vi "Period Curve from Matrix Signals.vi"(5 "S-G Polynomial Order":i32=3, 6 "Interpolation Method":i32(ring)=2 items=["nearest", "linear", "spline", "cubic Hermite", "Lagrange"], 7 "S-G Side Points":i32=15, 9 "first_discard_bins":dbl=100.0, 11 "Signals Matrix":T1) -> (0 "Not-Extended Period Length Curve":cluster{"yi":dbl[], "yi":dbl[]}(graph), 2 "Period Length Curve by  Fitting":dbl[](graph), 3 "Period Length Curve by Interpolation":dbl[](graph))   [LabVIEW 2014]
uses:
  <vilib>/Analysis/Matrix/Datatypes/RealMatrix.ctl
  <vilib>/Analysis/3filter.llb/Savitzky-Golay Filter (DBL).vi
  <vilib>/imath/engines/lvmath2/RunTimeEngine/RangeToken/NIMS_Range.vi
  <instcachedir>/0/NIMS_Range_9BCE657718DF4976A877346C61F22738.lvgen/NIMS_Range_9BCE657718DF4976A877346C61F22738_001.vi
  <vilib>/imathl/engines/lvmath/Functions/Error Handling/Create Error.vi
  <vilib>/imath/engines/lvmath2/RunTimeEngine/BuiltInFunctions/polyfit/NIMS_[2o]_polyfit.vi
  <vilib>/imath/engines/lvmath2/RunTimeEngine/ErrorHandling/NIMS_Error From Error Code.vi
  <vilib>/imath/engines/lvmath2/RunTimeEngine/BuiltInFunctions/polyval/NIMS_polyval(GV,GM).vi
  <instcachedir>/0/NIMS_polyval(GV,GM)_E12556DC54744E0C81968744501C4F35.lvgen/NIMS_polyval(GV,GM)_E12556DC54744E0C81968744501C4F35_002.vi
  <vilib>/imath/engines/lvmath2/RunTimeEngine/ArithmeticOperatorToken/NIMS_ArithmeticOperator_minus.vi
  <instcachedir>/0/NIMS_ArithmeticOperator_minus_39C0593E74DA4138ACA2AB742906488D.lvgen/NIMS_ArithmeticOperator_minus_39C0593E74DA4138ACA2AB742906488D_003.vi
  <vilib>/imath/engines/lvmath2/RunTimeEngine/NodeEndStatement/NIMS_NodeEndStatement_Output.vi
  <instcachedir>/0/NIMS_NodeEndStatement_Output_53EC0D466D134D7ABD903AC30B43404B.lvgen/NIMS_NodeEndStatement_Output_53EC0D466D134D7ABD903AC30B43404B_005.vi
  <vilib>/imath/engines/lvmath2/RunTimeEngine/ErrorHandling/NIMS_Finalize Error.vi
  <vilib>/imath/engines/lvmath2/RunTimeEngine/BuiltInFunctions/round/NIMS_round(DBL-V).vi
  <vilib>/imath/engines/lvmath2/RunTimeEngine/BuiltInFunctions/difference/NIMS_difference(GV,I32).vi
  <instcachedir>/0/NIMS_difference(GV,I32)_DC7351DCBCF840A8AE147F50EC2CE86E.lvgen/NIMS_difference(GV,I32)_DC7351DCBCF840A8AE147F50EC2CE86E_000.vi
  <vilib>/imath/engines/lvmath2/RunTimeEngine/BuiltInFunctions/size/NIMS_I32=size(GCol,I32).vi
  <instcachedir>/0/NIMS_I32=size(GCol,I32)_E76181316ED84D3E8F11BE44C7815EB0.lvgen/NIMS_I32=size(GCol,I32)_E76181316ED84D3E8F11BE44C7815EB0_000.vi
  <vilib>/imath/engines/lvmath2/RunTimeEngine/IndexRead/NIMS V(R2).vi
  <instcachedir>/0/NIMS V(R2)_C76619605A0E4E9F8B2FA9389712AC47.lvgen/NIMS V(R2)_C76619605A0E4E9F8B2FA9389712AC47_000.vi
  <vilib>/imath/engines/lvmath2/RunTimeEngine/ErrorHandling/NIMS_Create Error From Enums.vi
  <vilib>/imath/engines/lvmath2/RunTimeEngine/BuiltInFunctions/zeros/NIMS_M=zeros(I32).vi
  <vilib>/imath/engines/lvmath2/RunTimeEngine/RangeToken/NIMS_Range_R2 - Integer.vi
  <instcachedir>/0/NIMS_Range_R2 - Integer_2D1304BAF97744E0A293025746CBADFC.lvgen/NIMS_Range_R2 - Integer_2D1304BAF97744E0A293025746CBADFC_000.vi
  <vilib>/imath/engines/lvmath2/RunTimeEngine/CommandStatement/MC_CommandStatement_break.vi
  <vilib>/imath/engines/lvmath2/RunTimeEngine/IndexRead/NIMS V(S).vi
  <instcachedir>/0/NIMS V(S)_0488751826AF41519A22953C041130DC.lvgen/NIMS V(S)_0488751826AF41519A22953C041130DC_000.vi
  <vilib>/imath/engines/lvmath2/RunTimeEngine/IndexReplace/NIMS M(S)=S.vi
  <instcachedir>/0/NIMS M(S)=S_D871EE7B27E5455586ED06C330670F09.lvgen/NIMS M(S)=S_D871EE7B27E5455586ED06C330670F09_001.vi
  <vilib>/imath/engines/lvmath2/RunTimeEngine/IndexRead/NIMS M($,S).vi
  <instcachedir>/0/NIMS M($,S)_3E5749BBB62E49528D4765A77F1F6D98.lvgen/NIMS M($,S)_3E5749BBB62E49528D4765A77F1F6D98_000.vi
  <vilib>/imath/engines/lvmath2/RunTimeEngine/BuiltInFunctions/zeros/NIMS_M=zeros(I32,I32).vi
  <vilib>/imath/engines/lvmath2/RunTimeEngine/IndexRead/NIMS M(S,$).vi
  <instcachedir>/0/NIMS M(S,$)_F24F360562DE41D8BE234322A2E15C65.lvgen/NIMS M(S,$)_F24F360562DE41D8BE234322A2E15C65_000.vi
  <vilib>/imath/engines/lvmath2/RunTimeEngine/BuiltInFunctions/size/NIMS_I32=size(GRow,I32).vi
  <instcachedir>/0/NIMS_I32=size(GRow,I32)_4662369BBD5B4B51BF0F6B31B2927178.lvgen/NIMS_I32=size(GRow,I32)_4662369BBD5B4B51BF0F6B31B2927178_000.vi
  <vilib>/imath/engines/lvmath2/RunTimeEngine/BuiltInFunctions/size/NIMS_I32Row=size(GCol).vi
  <instcachedir>/0/NIMS_I32Row=size(GCol)_6F63159FA7824881BFA06400543D6D03.lvgen/NIMS_I32Row=size(GCol)_6F63159FA7824881BFA06400543D6D03_000.vi
  <vilib>/imath/engines/lvmath2/RunTimeEngine/IndexRead/NIMS M($,R2).vi
  <instcachedir>/0/NIMS M($,R2)_D9380E19261A4ADFB2D364AF6959C6EF.lvgen/NIMS M($,R2)_D9380E19261A4ADFB2D364AF6959C6EF_001.vi
  <vilib>/imath/engines/lvmath2/RunTimeEngine/ArithmeticOperatorToken/NIMS_ArithmeticOperator_plus.vi
  <instcachedir>/0/NIMS_ArithmeticOperator_plus_48D6EAACA5D645B09F7EC9C016C2DEA8.lvgen/NIMS_ArithmeticOperator_plus_48D6EAACA5D645B09F7EC9C016C2DEA8_004.vi
  <vilib>/imath/engines/lvmath2/RunTimeEngine/IndexReplace/NIMS M(S,$)=V.vi
  <instcachedir>/0/NIMS M(S,$)=V_8321FD9A786642FB877A2933E8B48D2A.lvgen/NIMS M(S,$)=V_8321FD9A786642FB877A2933E8B48D2A_000.vi
  <instcachedir>/0/NIMS_NodeEndStatement_Output_53EC0D466D134D7ABD903AC30B43404B.lvgen/NIMS_NodeEndStatement_Output_53EC0D466D134D7ABD903AC30B43404B_002.vi
  <instcachedir>/0/NIMS_Range_9BCE657718DF4976A877346C61F22738.lvgen/NIMS_Range_9BCE657718DF4976A877346C61F22738_000.vi
  <instcachedir>/0/NIMS_NodeEndStatement_Output_53EC0D466D134D7ABD903AC30B43404B.lvgen/NIMS_NodeEndStatement_Output_53EC0D466D134D7ABD903AC30B43404B_001.vi
  <vilib>/imath/engines/lvmath2/RunTimeEngine/BuiltInFunctions/vconcatmx/NIMS_vconcatmx.vi
  <instcachedir>/0/NIMS_vconcatmx_3F7EE7E265C34A1F815AF13176DC5310.lvgen/NIMS_vconcatmx_3F7EE7E265C34A1F815AF13176DC5310_000.vi
  <vilib>/Analysis/NI_AALBase.lvlib
  <vilib>/Analysis/NI_AAL_SigProc.lvlib
  <vilib>/gmath/NI_Gmath.lvlib
  <vilib>/Analysis/Matrix/NI_Matrix.lvlib
panel:
  # "Smoothing: Savitzky-Golay Parameters"
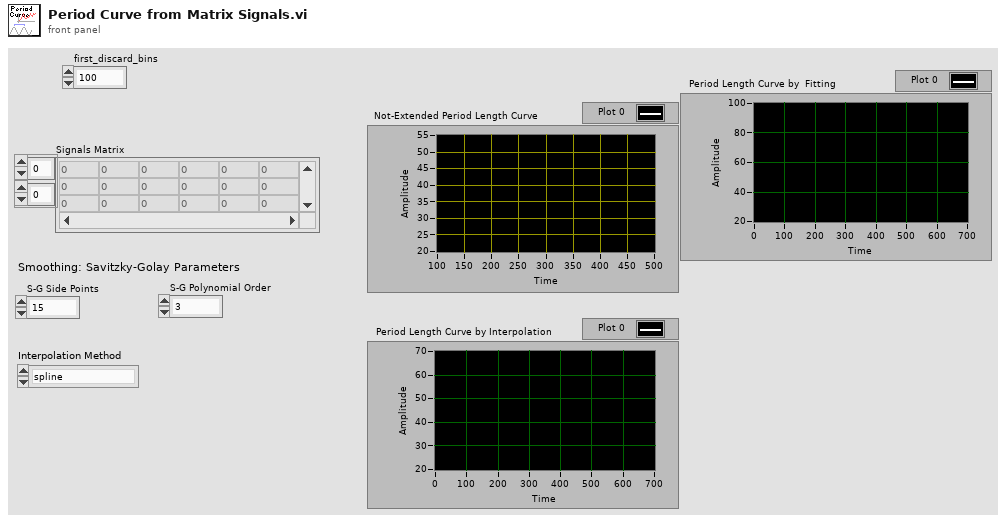
[diagram p1: front panel]
types:
  T1 = typedef "NI_Matrix.lvlib/RealMatrix.ctl" = dbl[][]
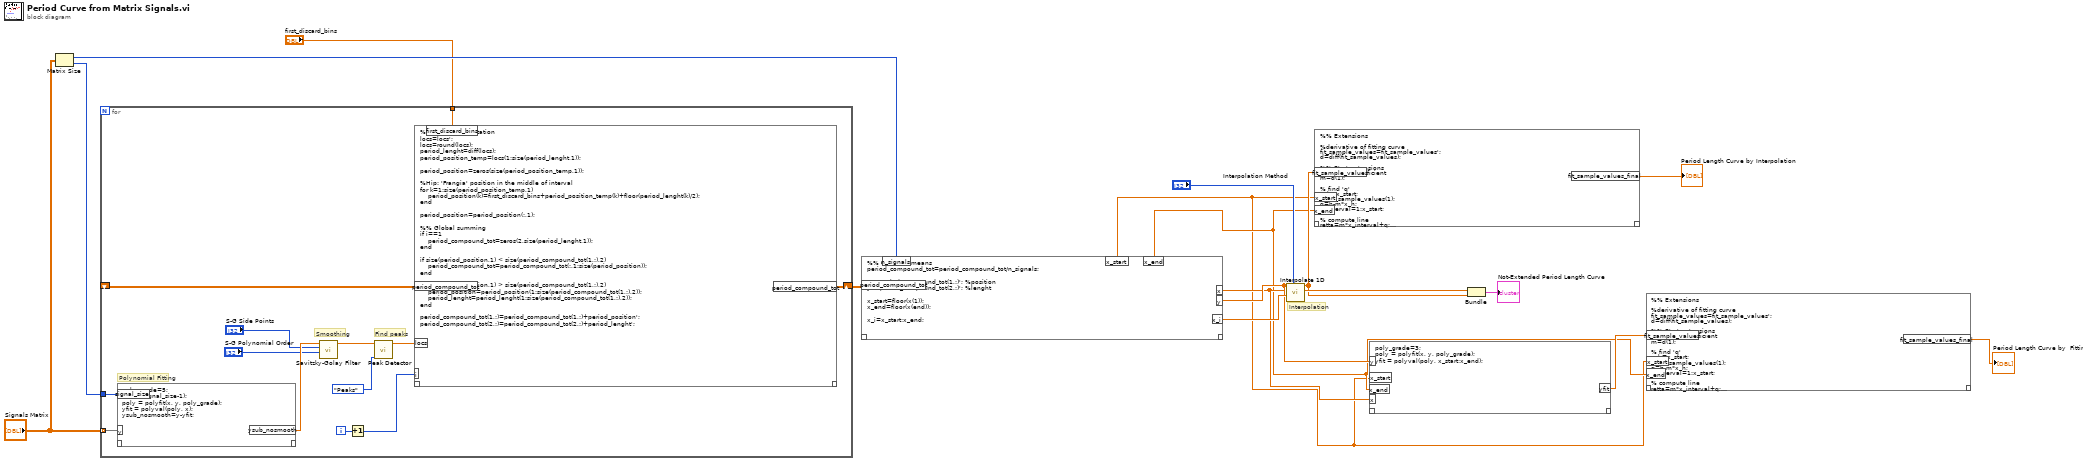
[diagram p0: block diagram]
diagram:
  # "Interpolation"
  n1 = Matrix Size(0:"Signals Matrix") -> (1:w13:i32, 2:w12:i32)
  n2 = for {
    tunnel: "Signals Matrix" -> [w26] mode=indexing
    shift-right: [w23] -> w17
    shift-left: _ -> [w22]
    tunnel: w12 -> [w21]
    tunnel: "first_discard_bins" -> [w18]
    i -> [w24]
    # "Find peaks"
    # "Smoothing"
    # "Polynomial Fitting"
    n3 = mathscript code="poly_grade=5;\nx = 0:(signal_size-1);\npoly = polyfit(x, y, poly_grade); \nyfit = polyval(poly, x); \nysub_nosmooth=y-yfit;"("signal_size"=w21, "y"=w26) -> ("ysub_nosmooth"=w30:dbl[])  [unwired: 1 in, 1 out]
    n4 = call-poly <vilib>:"Savitzky-Golay Filter.vi"("polynomial order"="S-G Polynomial Order", "side points"="S-G Side Points", "X"=w30) -> ("Filtered X"=w28:dbl[])  [unwired: 7 in, 1 out]
    n5 = Increment(x=w24) -> (x+1=w25:i32)
    n6 = call <vilib>:"Peak Detector.vi"("peaks/valleys"=enum32{"Peaks", "Valleys"}."Peaks", "X"=w28) -> ("Locations"=w27:dbl[])  [unwired: 5 in, 4 out]
    n7 = mathscript code="%% Period computation\nlocs=locs';\nlocs=round(locs);\nperiod_lenght=diff(locs);\nperiod_position_temp=locs(1:size(period_lenght,1)); \n\nperiod_position=zeros(size(period_position_temp,1));\n\n%Hip: 'Frangia' position in the middle of interval\nfor k=1:size(period_position_temp,1)\n    period_position(k)=first_discard_bins+period_position_temp(k)+floor(period_lenght(k)/2);\nend\n\nperiod_position=period_position(:,1);\n\n%% Global summing\nif i==1\n    period_compound_tot=zeros(2,size(period_lenght,1));\nend\n\nif size(period_position,1) < size(period_compound_tot(1,:),2)\n    period_compound_tot=period_compound_tot(:,1:size(period_position));\nend\n\nif size(period_position,1) > size(period_compound_tot(1,:),2)\n    period_position=period_position(1:size(period_compound_tot(1,:),2));\n    period_lenght=period_lenght(1:size(period_compound_tot(1,:),2));\nend\n\nperiod_compound_tot(1,:)=period_compound_tot(1,:)+period_position';\nperiod_compound_tot(2,:)=period_compound_tot(2,:)+period_lenght';"("locs"=w27, "first_discard_bins"=w18, "i"=w25, "period_compound_tot"=w22) -> ("period_compound_tot"=w23:dbl[][])  [unwired: 1 in, 1 out]
  }
  n8 = mathscript code="%% Compute means\nperiod_compound_tot=period_compound_tot/n_signals;\n\nx = period_compound_tot(1,:)'; %position\ny = period_compound_tot(2,:)'; %lenght\n\nx_start=floor(x(1));\nx_end=floor(x(end));\n\nx_i=x_start:x_end;"("period_compound_tot"=w17, "n_signals"=w13) -> ("x"=w5:dbl[], "y"=w6:dbl[], "x_start"=w1:dbl, "x_end"=w2:dbl, "x_i"=w7:dbl[])  [unwired: 1 in, 1 out]
  n9 = call <vilib>:"Interpolate 1D.vi"("method"="Interpolation Method", "xi"=w7, "X"=w5, "Y"=w6) -> ("xi used"=w15:dbl[], "yi"=w14:dbl[])  [unwired: 5 in, 1 out]
  n10 = mathscript code="%% Extensions\n\n%derivative of fitting curve\nfit_sample_values=fit_sample_values';\nd=diff(fit_sample_values);\n\n%% Start extensions\n% angular coefficient\nm=d(1);\n\n% find 'q'\nx_h=x_start;\nh=fit_sample_values(1);\nq=h-m*x_h;\nx_interval=1:x_start;\n\n% compute line\nretta=m*x_interval+q;\nretta=retta-(retta(end)-fit_sample_values(1));\nfit_sample_values_final=vertcat(retta(1:(end-1))',fit_sample_values);\n\n%% End extension\n% angular coefficient\nm=d(end);\n\n% find 'q'\nx_h=x_end;\nh=fit_sample_values(end);\nq=h-m*x_h;\nx_interval=x_end:625;\n\n% compute line\nretta_2=m*x_interval+q;\nretta_2=retta_2+(fit_sample_values(end)-retta_2(1));\nfit_sample_values_final=vertcat(fit_sample_values_final,retta_2(2:end)');\n\nfit_sample_values_final=fit_sample_values_final(:,1);"("fit_sample_values"=w14, "x_start"=w1, "x_end"=w2) -> ("fit_sample_values_final"=→"Period Length Curve by Interpolation":dbl[])  [unwired: 1 in, 1 out]
  n11 = mathscript code="poly_grade=3;\npoly = polyfit(x, y, poly_grade); \nyfit = polyval(poly, x_start:x_end);"("y"=w6, "x"=w5, "x_start"=w1, "x_end"=w2) -> ("yfit"=w4:dbl[])  [unwired: 1 in, 1 out]
  n12 = Bundle("xi used"=w15, "yi"=w14) -> (→"Not-Extended Period Length Curve":cluster{"xi used":dbl[], "yi":dbl[]})  [unwired: 1 in]
  n13 = mathscript code="%% Extensions\n\n%derivative of fitting curve\nfit_sample_values=fit_sample_values';\nd=diff(fit_sample_values);\n\n%% Start extensions\n% angular coefficient\nm=d(1);\n\n% find 'q'\nx_h=x_start;\nh=fit_sample_values(1);\nq=h-m*x_h;\nx_interval=1:x_start;\n\n% compute line\nretta=m*x_interval+q;\nretta=retta-(retta(end)-fit_sample_values(1));\nfit_sample_values_final=vertcat(retta(1:(end-1))',fit_sample_values);\n\n%% End extension\n% angular coefficient\nm=d(end);\n\n% find 'q'\nx_h=x_end;\nh=fit_sample_values(end);\nq=h-m*x_h;\nx_interval=x_end:625;\n\n% compute line\nretta_2=m*x_interval+q;\nretta_2=retta_2+(fit_sample_values(end)-retta_2(1));\nfit_sample_values_final=vertcat(fit_sample_values_final,retta_2(2:end)');\n\nfit_sample_values_final=fit_sample_values_final(:,1);"("fit_sample_values"=w4, "x_start"=w1, "x_end"=w2) -> ("fit_sample_values_final"=→"Period Length Curve by  Fitting":dbl[])  [unwired: 1 in, 1 out]
